vi "Omni-teste-Fast-2.vi"() -> ()   [LabVIEW 2012]
uses:
  <vilib>/Analysis/NI_AALBase.lvlib
panel:
  out "Waveform Chart":u32(graph)
  out "size(s)":i32
  out "variance":dbl format="%0.2f"
  out "standard deviation":dbl format="%0.2f"
  out "mean":dbl format="%0.2f"
  out "time":i32
  in  "stop":bool
  out "XY Graph":T1(graph)
  out "Length":i32
  in  "Correct Electrical Dark":bool
  in  "Integration Time (ms)":i32
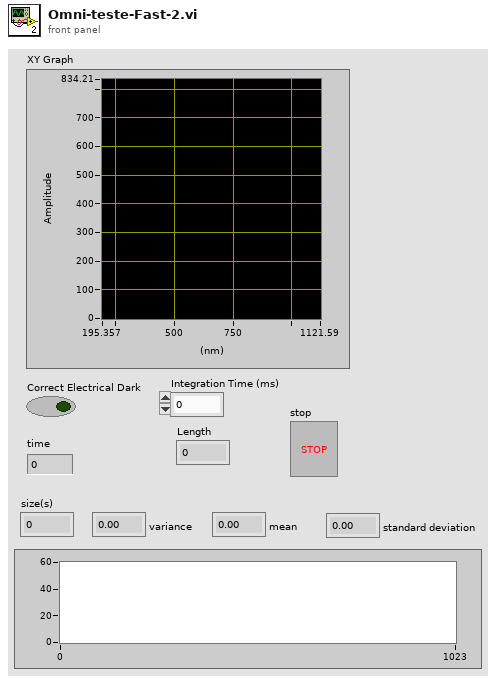
[diagram p1: front panel]
types:
  T1 = cluster{"WL Values":dbl[], "Spectrum Values":dbl[]}
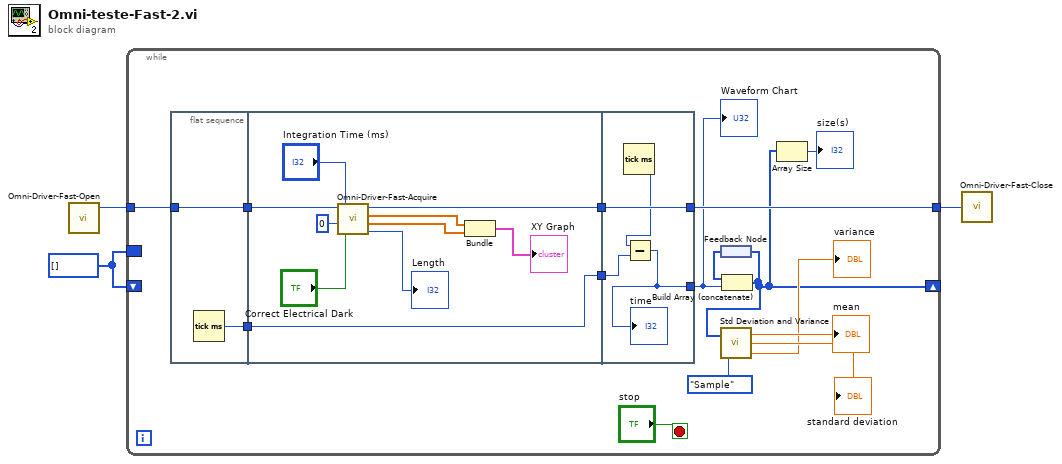
[diagram p0: block diagram]
diagram:
  w1 = u32[] []
  n1 = call "Omni-Driver-Fast-Open.vi"() -> ("Wrapper Out"=w3:u32)  [unwired: 4 in, 1 out]
  n2 = while {
    tunnel: w3 -> [w18]
    tunnel: [w17] -> w2
    shift-right: [w6] -> _
    shift-left: w1 -> [_]
    border: w1 -> [_]
    stop <- "stop" stop-if-true
    n3 = flat-sequence {
      tunnel: w18 -> [w20]
      tunnel: [w20] -> w15
      tunnel: [w19] -> w12
      tunnel: w15 -> [w30]
      tunnel: [w26] -> w14
      tunnel: [w21] -> w13
      tunnel: w12 -> [w21]
      tunnel: [w34] -> w17
      tunnel: w14 -> [w34]
      tunnel: w13 -> [w32]
      tunnel: [w31] -> w4
      frame #0 {
        n4 = Tick Count (ms)() -> (millisecond timer value=w19:u32)
      }
      frame #1 {
        n5 = call "Omni-Driver-Fast-Acquire.vi"("Correct Electrical Dark"="Correct Electrical Dark", "Spectrometer number"=0, "Integration Time (ms)"="Integration Time (ms)", "Wrapper"=w30) -> ("Length"=→"Length":i32, "Spectrum Values"=w24:dbl[], "WL Values"=w25:dbl[], "Wrapper Out"=w26:u32)
        n6 = Bundle("WL Values"=w25, "Spectrum Values"=w24) -> (→"XY Graph":T1)  [unwired: 1 in]
      }
      frame #2 {
        n7 = Tick Count (ms)() -> (millisecond timer value=w33:u32)
        n8 = Subtract(x=w33, y=w32) -> (x-y=w31:u32)
        "time" <- w31
      }
    }
    n9 = feedback #1() -> (w11:u32[])
    n10 = Build Array (concatenate)(w11, w4) -> (w6:u32[])
    n11 = feedback-in #1(w6) -> ()
    n12 = call <vilib>:"Std Deviation and Variance.vi"("X"=w6, "Weighting (Sample)"=enum16{"Sample", "Population"}."Sample") -> ("mean"=→"mean":dbl, "standard deviation"=→"standard deviation":dbl, "variance"=→"variance":dbl)
    n13 = Array Size(array=w6) -> (size(s)=→"size(s)":i32)
    "Waveform Chart" <- w4
  }
  n14 = call "Omni-Driver-Fast-Close.vi"("Wrapper In"=w2) -> ()  [unwired: 1 in]
